vi "Initialize Thread Settings.vi"(7 "component name":string, 8 "error in (no error)":errorcluster, 10 "Thread Configuration":refnum<class "Thread Configuration.lvclass">, 11 "GE Reflective Memory Transceiver in":refnum<class "GE Reflective Memory Transceiver.lvclass">) -> (0 "error out":errorcluster, 3 "GE Reflective Memory Transceiver out":refnum<class "GE Reflective Memory Transceiver.lvclass">)   [LabVIEW 2017, in "GE Reflective Memory.lvlib" / "GE Reflective Memory Transceiver.lvclass"]
uses:
  GE Reflective Memory Transceiver.lvclass
  DSF Core.lvlibp/Classes/Configuration/Core/Thread/Thread Configuration.lvclass
  Configurations/Thread/Thread Configuration.lvclass
  Configurations/Thread/Thread Configuration.lvclass/Thread Configuration.ctl
  GE Reflective Memory Transceiver.lvclass/GE Reflective Memory Transceiver.ctl
  DSF Core.lvlibp/Classes/Configuration/Core/Core Configuration.lvclass
  C:/Git/DSF/Components/DSF Core.lvlibp/Classes/Configuration/Core/Core Configuration.lvclass
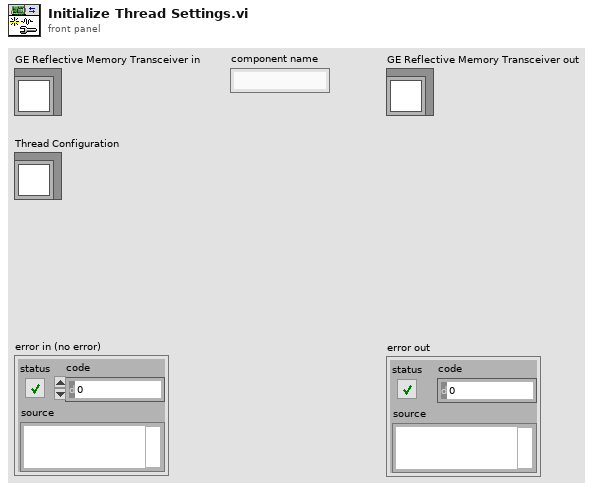
[diagram p1: front panel]
types:
  T1 = typedef "DSF Core.lvlibp/DSF Settings Info.ctl" = cluster{"component":string, "values":cluster{"key":string, "value":string}[]}
  T2 = typedef "GE 5565PIORC.lvclass/GE 5565PIORC.Typedef.DMA Wait Mode.ctl" = enum16{"Polling", "Interrupt"}
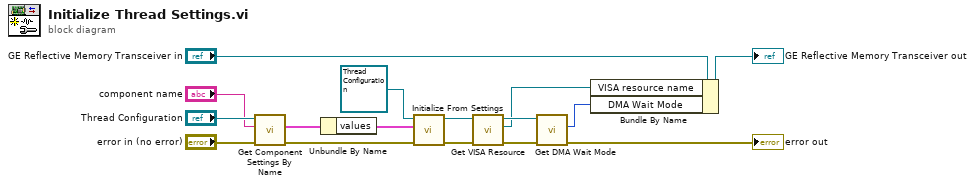
[diagram p0: block diagram]
diagram:
  n1 = call "Get Component Settings By Name.vi"("error in (no error)"="error in (no error)", "component name"="component name", "Runtime Configuration in"="Thread Configuration") -> ("error out"=w3:errorcluster, "component settings"=w2:T1)  [unwired: 6 in, 1 out]
  n2 = Unbundle By Name(w2) -> ("values"=w1:cluster{"key":string, "value":string}[])
  n3 = call-dynamic "Initialize From Settings.vi"("error in (no error)"=w3, "settings"=w1, "Thread Configuration in"=refnum<class "Thread Configuration.lvclass"> refnum ("GE Reflective Memory.lvlib:Thread Configuration.lvclass")) -> ("error out"=w13:errorcluster, "Thread Configuration out"=w12:refnum<class "Thread Configuration.lvclass">)  [unwired: 7 in]
  n4 = call "Get VISA Resource.vi"("error in (no error)"=w13, "Thread Configuration in"=w12) -> ("error out"=w10:errorcluster, "VISA Resource"=w8:refnum<visa-resource-name>, "Thread Configuration out"=w11:refnum<class "Thread Configuration.lvclass">)  [unwired: 7 in]
  n5 = call "Get DMA Wait Mode.vi"("error in (no error)"=w10, "Thread Configuration in"=w11) -> ("error out"=→"error out":errorcluster, "wait mode"=w9:T2)  [unwired: 7 in, 1 out]
  n6 = Bundle By Name(cluster="GE Reflective Memory Transceiver in", "VISA resource name"=w8, "DMA Wait Mode"=w9) -> (→"GE Reflective Memory Transceiver out":refnum<class "GE Reflective Memory Transceiver.lvclass">)
